vi "aoi_jpeg_rename.vi"() -> ()   [LabVIEW 2014]
panel:
  in  "Title":string
  in  "start":dbl format="%#_13g"
  in  "Folder path":path
  out "Filenames":string[](array[string])
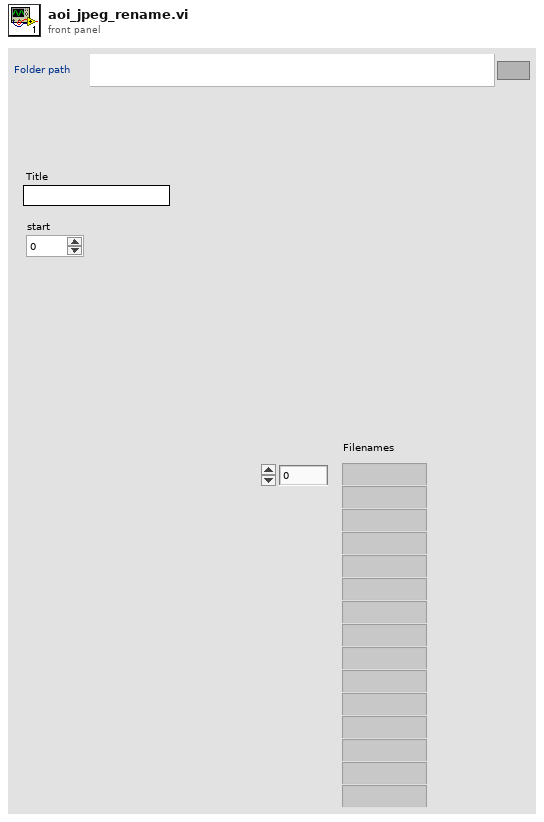
[diagram p1: front panel]
types:
  T1 = typedef "imagedata.ctl" = cluster{"image type":i32, "image depth":i32, "image":u8[], "mask":u8[], "colors":u32[], "Rectangle":cluster{"left":i16, "top":i16, "right":i16, "bottom":i16}}
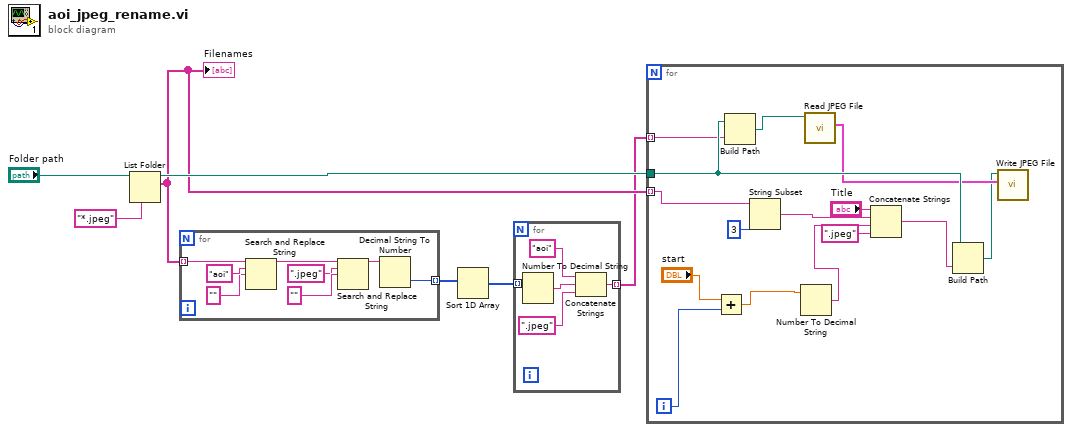
[diagram p0: block diagram]
diagram:
  n1 = List Folder(path="Folder path", pattern="*.jpeg") -> (path out=w5:path, filenames=w4:string[])  [unwired: 2 in, 2 out]
  "Filenames" <- w4
  n2 = for {
    tunnel: w4 -> [w15] mode=indexing
    tunnel: [w8] -> w3 mode=indexing
    n3 = Search and Replace String(input string=w15, search string="aoi", replace string="" ("replace string (\"\")")) -> (result string=w10:string)  [unwired: 5 in, 3 out]
    n4 = Search and Replace String(input string=w10, search string=".jpeg" ("replace string (\"\")"), replace string="" ("replace string (\"\")")) -> (result string=w9:string)  [unwired: 5 in, 3 out]
    n5 = Decimal String To Number(string=w9) -> (number=w8:i32)  [unwired: 2 in, 1 out]
  }
  n6 = Sort 1D Array(array=w3) -> (sorted array=w2:i32[])
  n7 = for {
    tunnel: w2 -> [w20] mode=indexing
    tunnel: [w16] -> w1 mode=indexing
    n8 = Number To Decimal String(number=w20) -> (decimal integer string=w17:string)  [unwired: 1 in]
    n9 = Concatenate Strings("aoi" ("search string"), w17, ".jpeg" ("string")) -> (w16:string)
  }
  n10 = for {
    tunnel: w4 -> [w26] mode=indexing
    tunnel: w5 -> [w27]
    tunnel: w1 -> [w22] mode=indexing
    i -> [w34]
    n11 = Add(x="start", y=w34) -> (x+y=w31:dbl)
    n12 = Build Path(base path=w27, name or relative path=w22) -> (appended path=w25:path)
    n13 = String Subset(string=w26, length (rest)=3 ("length (rest)")) -> (substring=w32:string)  [unwired: 1 in]
    n14 = Number To Decimal String(number=w31) -> (decimal integer string=w30:string)  [unwired: 1 in]
    n15 = call <vilib>:"Read JPEG File.vi"("path to JPEG file"=w25) -> ("image data"=w24:T1)  [unwired: 8 in, 2 out]
    n16 = Concatenate Strings("Title", w32, w30, ".jpeg" ("string")) -> (w28:string)
    n17 = Build Path(base path=w27, name or relative path=w28) -> (appended path=w23:path)
    n18 = call <vilib>:"Write JPEG File.vi"("image data"=w24, "path to JPEG file"=w23) -> ()  [unwired: 8 in, 2 out]
  }
